vi "RPI2 Check Linux Partition Size.vi"(8 "Error In":errorcluster, 10 "Warnings":T1[](array[typedef]), 11 "Install LV Data":T2={"SSH Session"=refnum, "Status Log"="", "Detailed Log"="", "Credentials"={"Hostname or IP"="192.168.7.2", "Username"="root", "Password"=""}, "Target Info"={"OS Version"="", "CPU"="", "Systemd Version"="", "Internet Access"=FALSE, "Device Type"="", "LV Installed Ver"="", "LV Available Ver"="", "LV Upgrade Available"=FALSE, "Hostname"="", "NIC Info"=[]}, "Reboot Required?"=FALSE}) -> (0 "Error Out":errorcluster, 2 "Warnings":T1[](array[typedef]), 3 "Install LV Data":T2={"SSH Session"=refnum, "Status Log"="", "Detailed Log"="", "Credentials"={"Hostname or IP"="192.168.7.2", "Username"="root", "Password"=""}, "Target Info"={"OS Version"="", "CPU"="", "Systemd Version"="", "Internet Access"=FALSE, "Device Type"="", "LV Installed Ver"="", "LV Available Ver"="", "LV Upgrade Available"=FALSE, "Hostname"="", "NIC Info"=[]}, "Reboot Required?"=FALSE})   [LabVIEW 2020, in "LMH-LINX.lvlib"]
uses:
  LMH-LINX.lvlib
  <vilib>/regexp/Match Regular Expression.xnode
  Target Compatibility Warnings.ctl
  RPI2 Expand File System.vi
  Target Info.ctl
  Install LV Data.ctl
  NIC Mode.ctl
  NIC Info.ctl
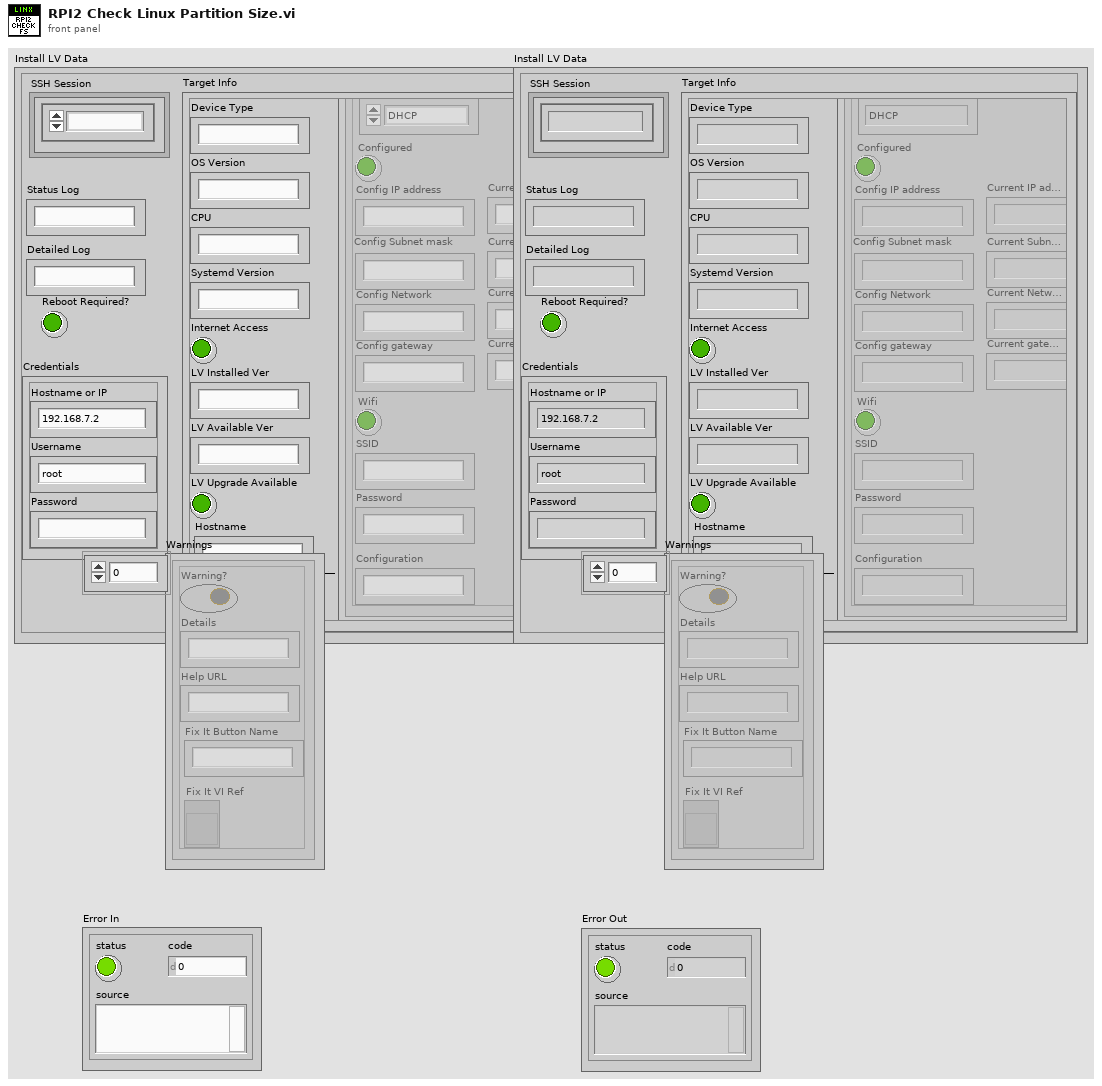
[diagram p1: front panel]
types:
  T1 = typedef "LMH-LINX.lvlib/Target Compatibility Warnings.ctl" = cluster{"Warning?":bool, "Details":string, "Help URL":string, "Fix It Button Name":string, "Fix It VI Ref":refnum<vi>}
  T2 = typedef "LMH-LINX.lvlib/Install LV Data.ctl" = cluster{"SSH Session":refnum<k1>, "Status Log":string, "Detailed Log":string, "Credentials":cluster{"Hostname or IP":string, "Username":string, "Password":string}, "Target Info":T3, "Reboot Required?":bool}
  T3 = typedef "LMH-LINX.lvlib/Target Info.ctl" = cluster{"OS Version":string, "CPU":string, "Systemd Version":string, "Internet Access":bool, "Device Type":string, "LV Installed Ver":string, "LV Available Ver":string, "LV Upgrade Available":bool, "Hostname":string, "NIC Info":T4[]}
  T4 = typedef "LMH-LINX.lvlib/NIC Info.ctl" = cluster{"Name":string, "NIC Mode":T5, "Configured":bool, "Config IP address":string, "Config Subnet mask":string, "Config Network":string, "Config gateway":string, "Wifi":bool, "SSID":string, "Password":string, "Configuration":string, "Current IP address":string, "Current Subnet mask":string, "Current gateway":string, "Current Network":string}
  T5 = typedef "LMH-LINX.lvlib/NIC Mode.ctl" = enum16{"DHCP", "Static", "Loopback"}
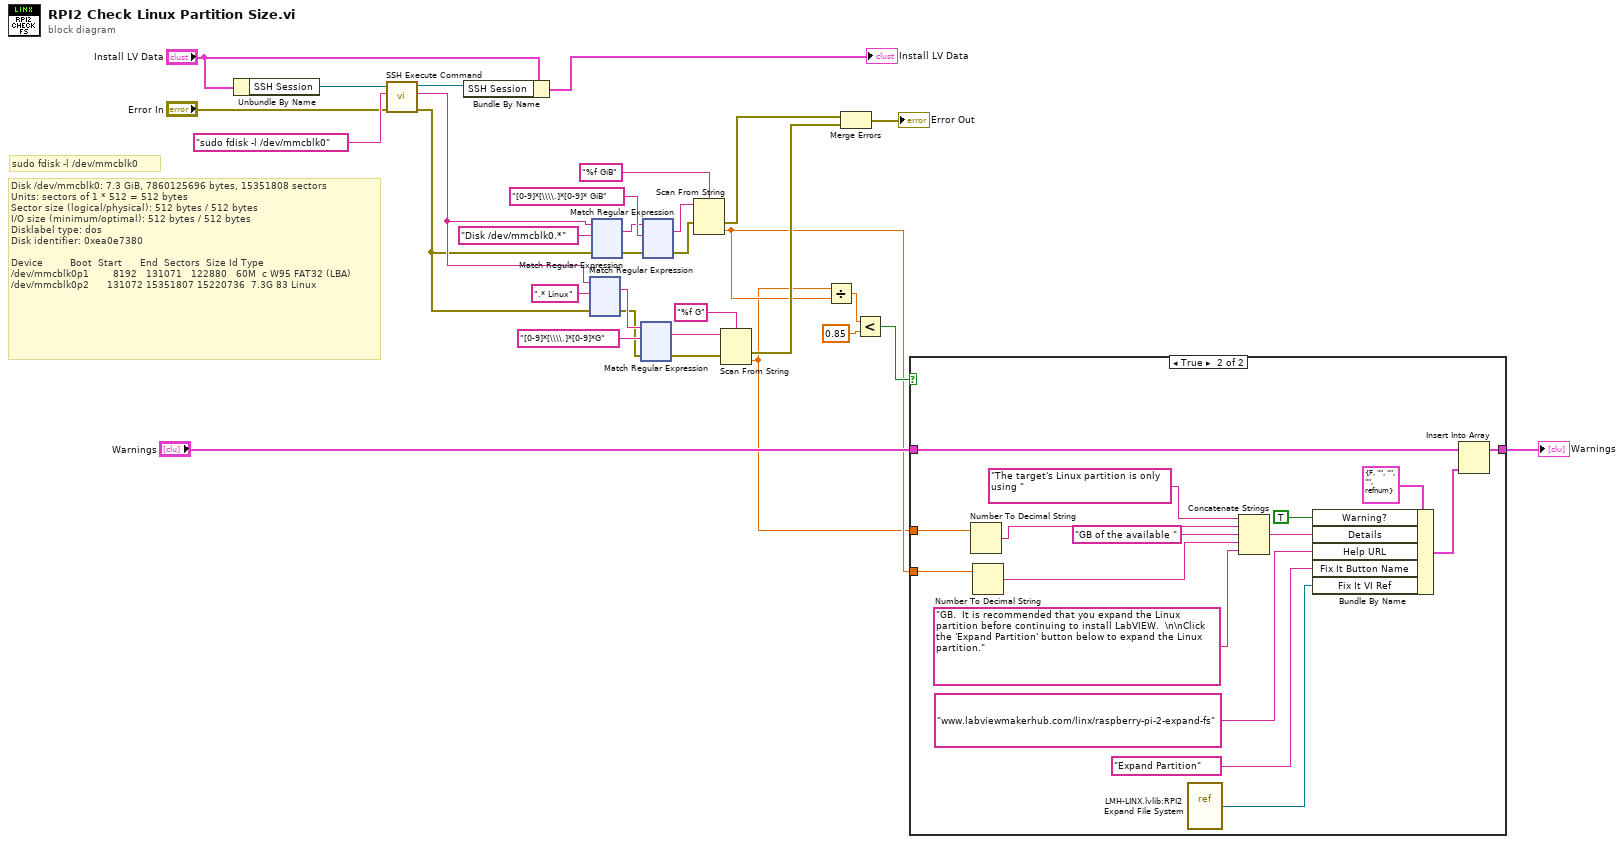
[diagram p0: block diagram]
diagram:
  # "sudo fdisk -l /dev/mmcblk0"
  # "Disk /dev/mmcblk0: 7.3 GiB, 7860125696 bytes, 15351808 sectors\nUnits: sectors of 1 * 512 = 512 bytes\nSector size (logical/physical): 512 bytes / 512 bytes\nI/O size (minimum/optimal): 512 bytes / 512 bytes\nDisklabel type: dos\nDisk identifier: 0xea0e7380\n\nDevice         Boot  Start      End  Sectors  Size Id Type\n/dev/mmcblk0p1        8192   131071   122880   60M  c W95 FAT32 (LBA)\n/dev/mmcblk0p2      131072 15351807 15220736  7.3G 83 Linux"
  n1 = Unbundle By Name("Install LV Data") -> ("SSH Session"=w32:refnum<k1>)
  n2 = call "SSH Execute Command.vi"("Error In"="Error In", "Command"="sudo fdisk -l /dev/mmcblk0", "SSH Session"=w32) -> ("Error Out"=w11:errorcluster, "Std Out"=w15:string, "SSH Session"=w29:refnum<k1>)  [unwired: 6 in]
  n3 = Bundle By Name(cluster="Install LV Data", "SSH Session"=w29) -> (→"Install LV Data":T2)
  n4 = xnode "Match Regular Expression"("input string"=w15, "regular expression"=".* Linux" ("String"), "error in"=w11) -> ("whole match"=w19:string, "error out"=w10:errorcluster)  [unwired: 3 in, 3 out]
  n5 = xnode "Match Regular Expression"("input string"=w15, "regular expression"="Disk /dev/mmcblk0.*" ("String"), "error in"=w11) -> ("whole match"=w21:string, "error out"=w25:errorcluster)  [unwired: 3 in, 3 out]
  n6 = xnode "Match Regular Expression"("input string"=w19, "regular expression"="[0-9]*[\\\\.]*[0-9]*G" ("String"), "error in"=w10) -> ("whole match"=w17:string, "error out"=w9:errorcluster)  [unwired: 3 in, 3 out]
  n7 = xnode "Match Regular Expression"("input string"=w21, "regular expression"="[0-9]*[\\\\.]*[0-9]* GiB" ("String"), "error in"=w25) -> ("whole match"=w22:string, "error out"=w12:errorcluster)  [unwired: 3 in, 3 out]
  n8 = Scan From String(format string="%f GiB", input string=w22, error in=w12) -> (error out=w7:errorcluster, output 1=w2:dbl)  [unwired: 2 in, 2 out]
  n9 = Scan From String(format string="%f G", input string=w17, error in=w9) -> (error out=w6:errorcluster, output 1=w1:dbl)  [unwired: 2 in, 2 out]
  n10 = Divide(x=w1, y=w2) -> (x/y=w14:dbl)
  n11 = Merge Errors(w7, w6) -> (→"Error Out":errorcluster)
  n12 = Less?(x=w14, y=0.85) -> (x < y?=w3:bool)
  n13 = case shown="True" w3 {
    tunnel: "Warnings" -> [w33 w44]
    tunnel: [w33 w43] -> w4
    tunnel: w1 -> [_ w42]
    tunnel: w2 -> [_ w36]
    frame False {
    }
    frame True {
      n14 = Number To Decimal String(number=w42) -> (decimal integer string=w41:string)  [unwired: 1 in]
      n15 = Number To Decimal String(number=w36) -> (decimal integer string=w39:string)  [unwired: 1 in]
      n16 = vi-ref "LMH-LINX.lvlib:RPI2 Expand File System.vi"() -> (w35:refnum<vi>)
      n17 = Concatenate Strings("The target's Linux partition is only using ", w41, "GB of the available " ("string"), w39, "GB.  It is recommended that you expand the Linux partition before continuing to install LabVIEW.  \n\nClick the 'Expand Partition' button below to expand the Linux partition." ("string")) -> (w45:string)
      n18 = Bundle By Name(cluster=T1 {"Warning?"=FALSE, "Details"="", "Help URL"="", "Fix It Button Name"="", "Fix It VI Ref"=refnum} ("Target Compatibility Warnings"), "Warning?"=TRUE ("Can Continue?"), "Details"=w45, "Help URL"="www.labviewmakerhub.com/linx/raspberry-pi-2-expand-fs" ("string"), "Fix It Button Name"="Expand Partition" ("string"), "Fix It VI Ref"=w35) -> (w46:T1)
      n19 = Insert Into Array(array=w44, new element=w46) -> (w43:T1[])  [unwired: 1 in]
    }
  }
  "Warnings" <- w4
